vi "Rd Wr telescope settings.vi"(7 "Telescope Name":string="Default", 8 "error in (no error)":errorcluster, 9 "Settings File":string="CC System Settings.json", 10 "Write? (F:Read)":bool, 11 "Telescope Settings":T1) -> (0 "error out":errorcluster, 3 "Telescope Settings":T1)   [LabVIEW 2021]
uses:
  PRIME Telescope/PRIME Telescope cluster Settings.ctl
  2e80df6d-94aa-46b9-8b94-ceea8c057880.vi
  659fb017-0e9f-42f9-b06e-930303f00cbc.vi
  <vilib>/JDP Science/JSONtext/Find Item.vi
  <vilib>/JDP Science/JSONtext/Next JSON Value.vi
  <vilib>/JDP Science/JSONtext/String Subset.vi
  <vilib>/JDP Science/JSONtext/Parsing/Advance past next JSON Value (inlined COPY).vi
  <vilib>/JDP Science/JSONtext/Parsing/Advance past whitespace.vi
  <vilib>/JDP Science/JSONtext/Parsing/Advance past String.vi
  <vilib>/JDP Science/JSONtext/Parsing/Advance past Number.vi
  <vilib>/JDP Science/JSONtext/Parsing/Advance past Line Ending.vi
  <vilib>/JDP Science/JSONtext/Parsing/Parse Full Path or Item Name.vi
  <vilib>/JDP Science/JSONtext/Parsing/Advance past Array.vi
  <vilib>/JDP Science/JSONtext/Parsing/Advance past Object.vi
  <vilib>/JDP Science/JSONtext/support/Error Cluster From Code.vi
  <vilib>/JDP Science/JSONtext/Offset/Find Item Locations by Path.vi
  <vilib>/JDP Science/JSONtext/JSON text to Variant.vi
  <vilib>/JDP Science/JSONtext/Variant to JSON Text.vi
  <vilib>/JDP Science/JSONtext/Set Item.vi
  <vilib>/JDP Science/JSONtext/LVClass Serializer/JSONtext LVClass Serializer.lvclass
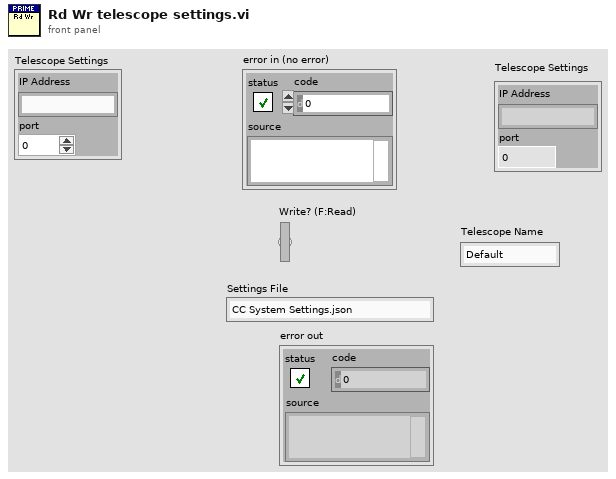
[diagram p1: front panel]
types:
  T1 = typedef "PRIME Telescope cluster Settings.ctl" = cluster{"IP Address":string, "port":u16}
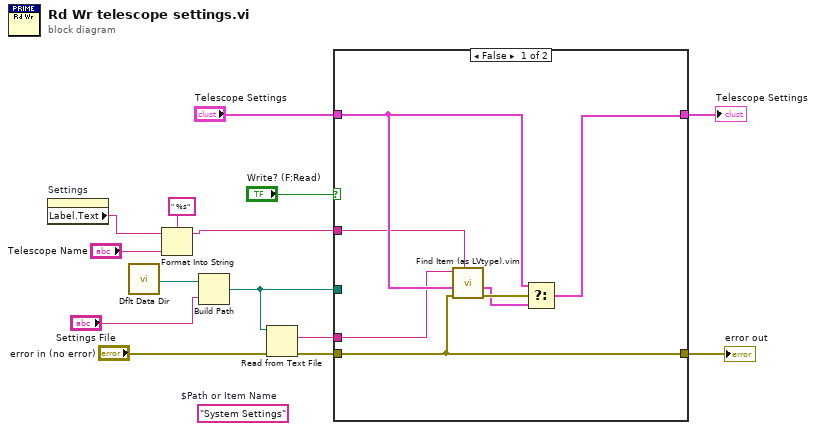
[diagram p0: block diagram]
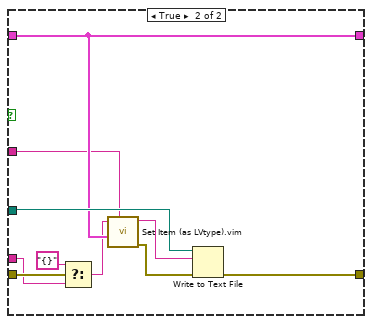
[diagram p2: hidden frame]
diagram:
  (unwired) "System Settings"  # $Path or Item Name
  n1 = property on="Settings" class="Clust (strict)"() -> ("Label.Text"=w2:string)  [unwired: 2 in, 2 out]
  n2 = call <vilib>:"Dflt Data Dir.vi"() -> ("App:Default Data Directory"=w11:path)
  n3 = Format Into String(format string=" %s", initial string=w2, "Telescope Name") -> (resulting string=w1:string)  [unwired: 1 in, 1 out]
  n4 = Build Path(base path=w11, name or relative path="Settings File") -> (appended path=w5:path)
  n5 = Read from Text File(file (use dialog)=w5, error in="error in (no error)") -> (text=w6:string, error out=w7:errorcluster)  [unwired: 2 in, 2 out]
  n6 = case shown="False" "Write? (F:Read)" {
    tunnel: w7 -> [w16 w27]
    tunnel: "Telescope Settings" -> [w20 w29]
    tunnel: w5 -> [_ w31]
    tunnel: [w16 w30] -> w10
    tunnel: [w21 w29] -> w9
    tunnel: w6 -> [w17 w25]
    tunnel: w1 -> [w15 w22]
    frame False {
      n7 = call "Find Item (as LVtype).vim"("$Path or Item Name"=w15, "error in (no error)"=w16, "Data Type and Default Value"=w20, "JSON"=w17) -> ("error out"=w19:errorcluster, "Data"=w18:T1)  [unwired: 4 in, 2 out]
      n8 = Select(t=w20, s=w19, f=w18) -> (s? t:f=w21:T1)
    }
    frame True {
      n9 = Select(t="{}" ("JSON"), s=w27, f=w25) -> (s? t:f=w24:string)
      n10 = call "Set Item (as LVtype).vim"("$Path or Item Name"=w22, "Anything"=w29, "JSON"=w24) -> ("error out"=w23:errorcluster, "<JSON>"=w28:string)  [unwired: 5 in, 1 out]
      n11 = Write to Text File(file (use dialog)=w31, text=w28, error in=w23) -> (error out=w30:errorcluster)  [unwired: 1 in, 2 out]
    }
  }
  "error out" <- w10
  "Telescope Settings" <- w9
